vi "E700-Sequence.vi"(1 "Direction Switch":bool, 5 "Rotation Instance":refnum<class "Modbus Master.lvclass">, 11 "error in (no error)":errorcluster, 12 "Time (mS) - Seq 1":u32 caption="Time (mS)" max=60 step=1, 13 "Vertical Frequencey Setting (Hz) - Seq 1":dbl caption="Vertical Frequencey Setting (Hz)" max=60.0 step=1.0, 14 "Rotational Frequencey Setting (Hz) - Seq 1":dbl caption="Rotational Frequencey Setting (Hz)" max=60.0 step=1.0) -> (15 "error out":errorcluster)   [LabVIEW 2020]
uses:
  <vilib>/NI/Modbus Library/API/Master/Modbus Master.lvclass
  C:/Program Files (x86)/National Instruments/LabVIEW 2020/vi.lib/NI/Modbus Library/API/Modbus API.lvclass
  <vilib>/NI/Modbus Library/API/Modbus API.lvclass/Modbus API.ctl
  <vilib>/NI/Modbus Library/Transmission Data Unit/Transmission Data Unit.lvclass/Transmission Data Unit.ctl
  <vilib>/NI/Modbus Library/Transmission Data Unit/Write Unit ID.vi
  <vilib>/NI/Modbus Library/API/Read Transmission Data Unit.vi
  <vilib>/NI/Modbus Library/API/Write Transmission Data Unit.vi
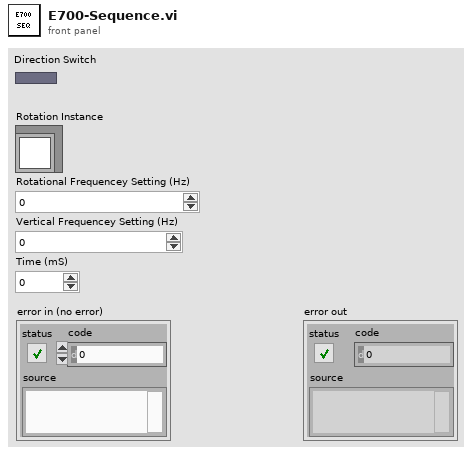
[diagram p1: front panel]
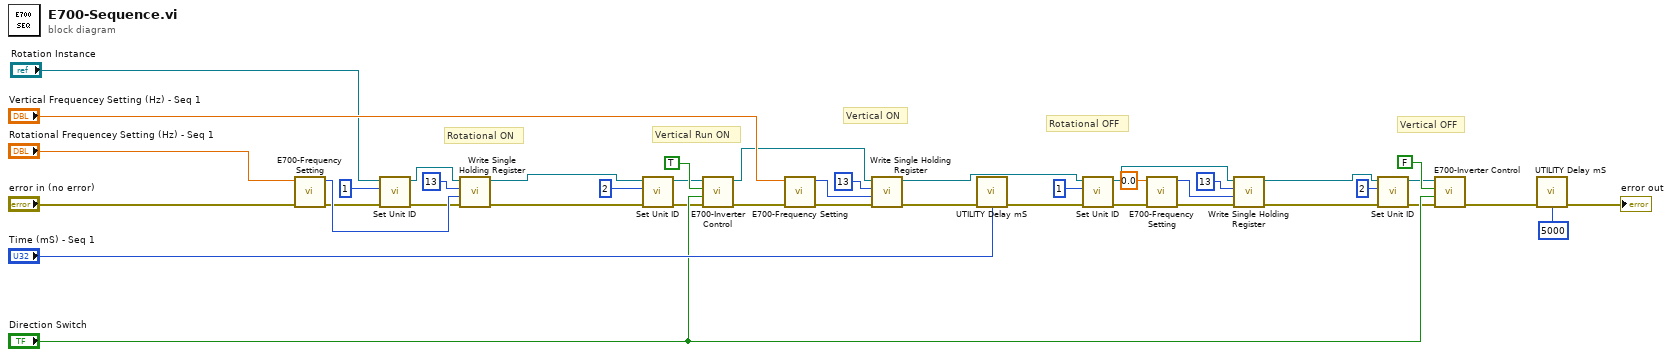
[diagram p0: block diagram]
diagram:
  # "Vertical Run ON"
  # "Vertical OFF"
  # "Vertical ON"
  # "Rotational OFF"
  # "Rotational ON"
  n1 = call "E700-Frequency Setting.vi"("error in (no error)"="error in (no error)", "Frequencey Setting (Hz)"="Rotational Frequencey Setting (Hz) - Seq 1") -> ("error out"=w23:errorcluster, "Set Value"=w38:u16)  [unwired: 8 in]
  n2 = call <vilib>:"Set Unit ID.vi"("error in"=w23, "unit ID"=u8 1, "Modbus master in"="Rotation Instance") -> ("error out"=w22:errorcluster, "Modbus master out"=w19:refnum<class "Modbus Master.lvclass">)  [unwired: 7 in]
  n3 = call-dynamic "Write Single Holding Register.vi"("error in"=w22, "register to write"=w38, "address"=u16 13, "Modbus master in"=w19) -> ("error out"=w17:errorcluster, "Modbus master out"=w15:refnum<class "Modbus Master.lvclass">)  [unwired: 6 in]
  n4 = call <vilib>:"Set Unit ID.vi"("error in"=w17, "unit ID"=u8 2, "Modbus master in"=w15) -> ("error out"=w16:errorcluster, "Modbus master out"=w14:refnum<class "Modbus Master.lvclass">)  [unwired: 7 in]
  n5 = call "E700-Inverter Control.vi"("error in (no error)"=w16, "Direction Switch"="Direction Switch", "ON/OFF - Switch"=TRUE, "Modbus Master in"=w14) -> ("error out"=w28:errorcluster, "Modbus Master out"=w26:refnum<class "Modbus Master.lvclass">)  [unwired: 6 in]
  n6 = call "E700-Frequency Setting.vi"("error in (no error)"=w28, "Frequencey Setting (Hz)"="Vertical Frequencey Setting (Hz) - Seq 1") -> ("error out"=w36:errorcluster, "Set Value"=w39:u16)  [unwired: 8 in]
  n7 = call-dynamic "Write Single Holding Register.vi"("error in"=w36, "register to write"=w39, "address"=u16 13, "Modbus master in"=w26) -> ("error out"=w37:errorcluster, "Modbus master out"=w10:refnum<class "Modbus Master.lvclass">)  [unwired: 6 in]
  n8 = call "UTILITY Delay mS.vi"("Error In"=w37, "milliseconds to wait"="Time (mS) - Seq 1") -> ("Error Out"=w12:errorcluster)  [unwired: 13 in]
  n9 = call <vilib>:"Set Unit ID.vi"("error in"=w12, "unit ID"=u8 1, "Modbus master in"=w10) -> ("error out"=w11:errorcluster, "Modbus master out"=w9:refnum<class "Modbus Master.lvclass">)  [unwired: 7 in]
  n10 = call "E700-Frequency Setting.vi"("error in (no error)"=w11, "Frequencey Setting (Hz)"=0.0) -> ("error out"=w33:errorcluster, "Set Value"=w32:u16)  [unwired: 8 in]
  n11 = call-dynamic "Write Single Holding Register.vi"("error in"=w33, "register to write"=w32, "address"=u16 13, "Modbus master in"=w9) -> ("error out"=w7:errorcluster, "Modbus master out"=w5:refnum<class "Modbus Master.lvclass">)  [unwired: 6 in]
  n12 = call <vilib>:"Set Unit ID.vi"("error in"=w7, "unit ID"=u8 2, "Modbus master in"=w5) -> ("error out"=w6:errorcluster, "Modbus master out"=w4:refnum<class "Modbus Master.lvclass">)  [unwired: 7 in]
  n13 = call "E700-Inverter Control.vi"("error in (no error)"=w6, "Direction Switch"="Direction Switch", "ON/OFF - Switch"=FALSE, "Modbus Master in"=w4) -> ("error out"=w3:errorcluster)  [unwired: 6 in, 1 out]
  n14 = call "UTILITY Delay mS.vi"("Error In"=w3, "milliseconds to wait"=u32 5000) -> ("Error Out"=→"error out":errorcluster)  [unwired: 13 in]
